vi "feedback(Host)_PIDXYZ_laserPID_COMTEMP.vi"(5 "RIO Device":T2="RIO0") -> ()   [LabVIEW 2018]
doc: "This VI will will initialize the FPGA VI and then continually read and convert single point values from 4 channels of an analog input module."
uses:
  <vilib>/userdefined/High Color/nirio_resource_hc.ctl
  <vilib>/rvi/Analysis/host/Butterworth/config/Butterworth Filter Order.ctl
  <vilib>/rvi/Analysis/host/Butterworth/config/Butterworth Filter Type.ctl
  <vilib>/FPGAPlugInAG/PXIe-7856R/niLvFpga_Open_PXIe-7856R.vi
  <vilib>/FPGAPlugInAG/PXIe-7856R/niLvFpga_Run_PXIe-7856R.vi
  <vilib>/Utility/error.llb/Error Cluster From Error Code.vi
  <vilib>/rvi/errors/niLvFpgaAdjustHostInterfaceError.vi
  <vilib>/rvi/Analysis/host/Butterworth/config/BwScaledCoefficients.vi
  <vilib>/rvi/Analysis/host/Notch/config/NotchScaledCoefficients.vi
  <vilib>/Utility/file.llb/Read From Spreadsheet File (I64).vi
  <vilib>/FPGAPlugInAG/PXIe-7856R/niLvFpga_Close_PXIe-7856R.vi
  <vilib>/rvi/interface/nirviOpenFPGA/nirviOpenFPGA.xnode
  FPGA Bitfiles/Microspherefeedb_FPGATarget2_(FPGA)PIDXYZ_reset_voltage.lvbitx
  <vilib>/rvi/interface/nirviMethod/nirviMethod.xnode
  <vilib>/rvi/interface/nirviReadWriteControl/nirviReadWriteControl.xnode
  <vilib>/rvi/Analysis/host/Butterworth/XNode/ButterworthCoefficients.xnode
  <vilib>/rvi/Analysis/host/Notch/XNode/NotchCoefficients.xnode
  <vilib>/rvi/interface/nirviCloseFPGA/nirviCloseFPGA.xnode
  <vilib>/rvi/Analysis/host/Public/NI_FpgaMspHost.lvlib
  NiFpgaLv.dll
panel:
  in  "Reset voltage":bool
  in  "If revert AO4 and AO5":bool
  in  "notch Q factor2 y":dbl=1.27
  in  "notch frequency2 y":dbl=265.5
  in  "If scan frequency (AO6 and AO7)?":bool
  in  "Amplitude AO7":i16
  in  "Amplitude AO6":i16
  in  "Amplitude AO5":i16
  in  "Amplitude AO4":i16
  in  "reset AO7":bool=TRUE
  in  "frequency AO7(Hz)":dbl=200000.0
  in  "phase offset AO7":fxp<+,32,0>
  in  "reset AO6":bool=TRUE
  in  "frequency AO6(Hz)":dbl=100000.0
  in  "phase offset AO6":fxp<+,32,0>=0.75
  in  "reset AO5":bool=TRUE
  in  "frequency AO5(Hz)":dbl=87.0
  in  "phase offset AO5":fxp<+,32,0>
  in  "reset AO4":bool=TRUE
  in  "frequency AO4(Hz)":dbl
  in  "phase offset AO4":fxp<+,32,0>
  in  "notch Q factor1 y":dbl=1.27
  in  "notch Q factor x":dbl=5.0
  in  "notch frequency1 y":dbl=572.4
  in  "notch frequency x":dbl=1000.0
  out "accum out z2":dbl(graph)
  out "accum out z1":dbl(graph)=1111.0
  in  "Reset x accum":bool=TRUE
  in  "Reset y accum":bool=TRUE
  in  "Reset z accum":bool=TRUE
  in  "Big Number":sgl=10000.0
  in  "amplitude_sine_EOM (V)":sgl
  in  "Freqency_sine_EOM (Hz)":sgl
  in  "Cluster":T1={"activate COMx"=FALSE, "activate  COMy"=FALSE, "activate COMz"=FALSE, "frequency (kHz)"=0.001500000013038516, "duty cycle (periods)"=0.10000000009313226, "offset"=8192, "amplitude"=8192, "Pz?"=FALSE, "Y_emergency_threshould"=23000, "X_emergency_threshould"=23000, "No_integral_Gain"=FALSE}
  in  "LP FF Z before":dbl=5000.0
  in  "LP FF Y before":dbl=5000.0
  in  "LP FF X Before":dbl=5000.0
  in  "LP FF Z":dbl=4200.0
  in  "LP FF Y":dbl=1300.0
  in  "LP FF X":dbl=1300.0
  in  "Lower lim Y before":fxp<+/-,16,16>=-150.0
  in  "Upper lim Y before":fxp<+/-,16,16>=150.0
  in  "Lower lim X before":fxp<+/-,16,16>=-15000.0
  in  "Upper lim X before":fxp<+/-,16,16>=15000.0
  in  "?":u16(ring)=2 items=["Both", "AOD", "Bead"]
  in  "?":u16(ring)=2 items=["Both", "AOD", "Bead"]
  out "Tot feedback + DC, Z":i16(graph)=5000
  out "Individual feedback, Z":cluster{"fb_0":i16, "fb_d0":i16}(graph)
  out "AI 2":cluster{"AI1":i16, "AI4":i16}(graph)={"AI1"=-2580, "AI4"=-2580}
  in  "Use PID Y before":bool
  in  "Use PID X before":bool
  in  "Ig Y before":fxp<+/-,24,-4>
  in  "Dg Y before":fxp<+/-,24,12>
  in  "Pg Y before":fxp<+/-,24,12>
  in  "Ig X before":fxp<+/-,24,-4>
  in  "Dg X before":fxp<+/-,24,12>
  in  "Pg X before":fxp<+/-,24,12>
  in  "Y before setpoint":i16
  in  "X before setpoint":i16
  in  "dg band X before":fxp<+/-,24,12>
  in  "dg band Y before":fxp<+/-,24,12>
  in  "hp freq X band before":dbl=5000.0
  in  "lp freq X band before":dbl=5000.0
  in  "hp freq X before":dbl=5000.0
  in  "lp freq X before":dbl=5000.0
  in  "hp freq Y band before":dbl=5000.0
  in  "lp freq Y band before":dbl=5000.0
  in  "hp freq Y before":dbl=5000.0
  in  "lp freq Y before":dbl=5000.0
  out "EOM_amplitude_out":dbl=-9.299359169972536
  in  "EOM_offset (-10 to 10 V)":dbl
  in  "EOM_amplitude (-10 to 10 V)":dbl=-9.3
  in  "EOM_threshold (0 to 1), (2*thr - 1)*ampli":dbl
  in  "EOM reset":bool
  in  "hp freq band Z before":dbl=5000.0
  in  "lp freq band Z before":dbl=5000.0
  in  "dg band Z before":fxp<+/-,24,12>
  in  "hp freq bandZ":dbl=49.0
  in  "lp freq bandZ":dbl=45.0
  in  "dg band Z":fxp<+/-,24,12>
  in  "dg band Y":fxp<+/-,24,12>
  in  "hp freq bandY":dbl=5000.0
  in  "lp freq bandY":dbl=5000.0
  in  "hp freq bandX":dbl=5000.0
  in  "lp freq bandX":dbl=5000.0
  in  "dg band X":fxp<+/-,24,12>
  in  "Pg Y":fxp<+/-,24,12>
  in  "Ig Y":fxp<+/-,24,-4>=8.009374141693115e-07
  in  "Pg X":fxp<+/-,24,12>
  in  "Ig X":fxp<+/-,24,-4>=-8.009374141693115e-07
  in  "End value arb (ch1)":fxp<+/-,32,16>
  in  "Step arb (ch1)":fxp<+/-,32,16>=0.100006103515625
  in  "Arb gain (Z)":fxp<+/-,24,12>
  in  "z arb scale":fxp<+/-,33,17>
  in  "ramp arb drive":bool
  in  "End value arb (ch0)":fxp<+/-,32,16>
  in  "Step arb (ch0)":fxp<+/-,32,16>
  in  "Delay Time (s) arb":dbl=0.001 caption="Delay Time (s)"
  in  "Buffer file path":path=path "C:/Users/yalem/GitHub/Documents/Optlev/scriptssinx_buffer.txt"
  in  "Write data to buffers":bool
  in  "Arb steps per cycle":u16=2
  in  "Arb gain (Y)":fxp<+/-,24,12>
  in  "Arb gain (X)":fxp<+/-,24,12>
  in  "Z before setpoint":i16
  in  "Upper lim Z before":fxp<+/-,16,16>=9999.0
  in  "Lower lim Z before":fxp<+/-,16,16>=-10000.0
  in  "hp freq Z before":dbl=5000.0
  in  "lp freq Z before":dbl=5000.0
  in  "Use PID Z before":bool
  in  "hp freq Y":dbl=400.0
  in  "hp freq X":dbl=400.0
  in  "lp freq X":dbl=200.0
  in  "DC offset X":i16=23000
  in  "Lower lim X":fxp<+/-,16,16>=-15000.0
  in  "Upper lim X":fxp<+/-,16,16>=15000.0
  in  "Dg X":fxp<+/-,24,12>
  in  "X setpoint":i16
  in  "change pars":bool
  in  "hp freq Z":dbl=4200.0
  in  "lp freq Y":dbl=200.0
  in  "lp freq Z":dbl=4200.0
  in  "ramp power":bool
  in  "End value power":i16=3000
  in  "Step power":i16=30
  in  "Delay Time (s) power":dbl=0.05 caption="Delay Time (s)"
  in  "Count(usec)":u32=10
  in  "?":u16(ring)=2 items=["Both", "AOD", "Bead"]
  in  "?":u16(ring)=2 items=["Both", "AOD", "Bead"]
  in  "?":u16(ring)=2 items=["Both", "AOD", "Bead"]
  in  "?":u16(ring)=2 items=["Both", "AOD", "Bead"]
  in  "Pg Z before":fxp<+/-,24,12>
  in  "Ig Z before":fxp<+/-,24,-4>
  in  "Dg Z before":fxp<+/-,24,12>
  in  "Ig Z":fxp<+/-,24,-4>=2.0116567611694336e-07
  in  "DC offset Z":i16=25000
  in  "Lower lim Z":fxp<+/-,16,16>=-22500.0
  in  "Upper lim Z":fxp<+/-,16,16>=23000.0
  in  "Dg Z":fxp<+/-,24,12>
  in  "Pg Z":fxp<+/-,24,12>
  in  "Z setpoint":i16=-3700
  in  "change pars 2":bool
  in  "change pars 1":bool
  in  "DC offset Y":i16=15000
  in  "Lower lim Y":fxp<+/-,16,16>=-20000.0
  in  "Upper lim Y":fxp<+/-,16,16>=20000.0
  in  "Dg Y":fxp<+/-,24,12>
  in  "Y setpoint":i16
  out "Tot feedback + DC, Y":i16(graph)=15000
  out "Individual feedback, Y":cluster{"fb_0":i16, "fb_d0":i16}(graph)
  out "AI1":cluster{"AI1":i16, "AI4":i16}(graph)={"AI1"=678, "AI4"=678}
  out "Tot feedback + DC, X":i16(graph)=23000
  out "Individual feedback, X":cluster{"fb_0":i16, "fb_d0":i16}(graph)
  out "AI0":cluster{"AI0":i16, "AI3":i16}(graph)={"AI0"=32295, "AI3"=32295}
  in  "stop":bool
  # "FPGA feedback GUI"
  # "Bead arbitrary drive:"
  # "PID controls, X (ch 0):"
  # "Bead feedback:"
  # "PID controls, Y (ch 1):"
  # "Bead feedback:"
  # "Rotation Control"
  # "AO6: Front\nAO7: Window\nAO4: Back\nAO5: Top"
  # "(mV)"
  # "Phase is in unit of periods"
  # "PID controls, Z (ch 2):"
  # "Bead feedback:"
  # "AOD feeback:"
types:
  T1 = cluster{"activate COMx":bool, "activate  COMy":bool, "activate COMz":bool, "frequency (kHz)":fxp<+,32,0>, "duty cycle (periods)":fxp<+,32,0>, "offset":i16, "amplitude":i16, "Pz?":bool, "Y_emergency_threshould":i16, "X_emergency_threshould":i16, "No_integral_Gain":bool}
  T2 = typedef "nirio_resource_hc.ctl" = tag
  T3 = cluster{"AI X plot":i16, "AI X before chamber plot":i16}
  T4 = cluster{"AI X before chamber plot":i16, "AI X before chamber plot":i16}
  T5 = cluster{"fb X plot":i16, "fb X before chamber plot":i16}
  T6 = cluster{"fb X before chamber plot":i16, "fb X before chamber plot":i16}
  T7 = cluster{"AI Y plot":i16, "AI Y before chamber plot":i16}
  T8 = cluster{"AI Y before chamber plot":i16, "AI Y before chamber plot":i16}
  T9 = cluster{"fb Y plot":i16, "fb Y before chamber plot":i16}
  T10 = cluster{"fb Y before chamber plot":i16, "fb Y before chamber plot":i16}
  T11 = cluster{"AI Z plot":i16, "AI Z before chamber plot":i16}
  T12 = cluster{"AI Z before chamber plot":i16, "AI Z before chamber plot":i16}
  T13 = cluster{"fb Z plot":i16, "fb Z before chamber plot":i16}
  T14 = cluster{"fb Z before chamber plot":i16, "fb Z before chamber plot":i16}
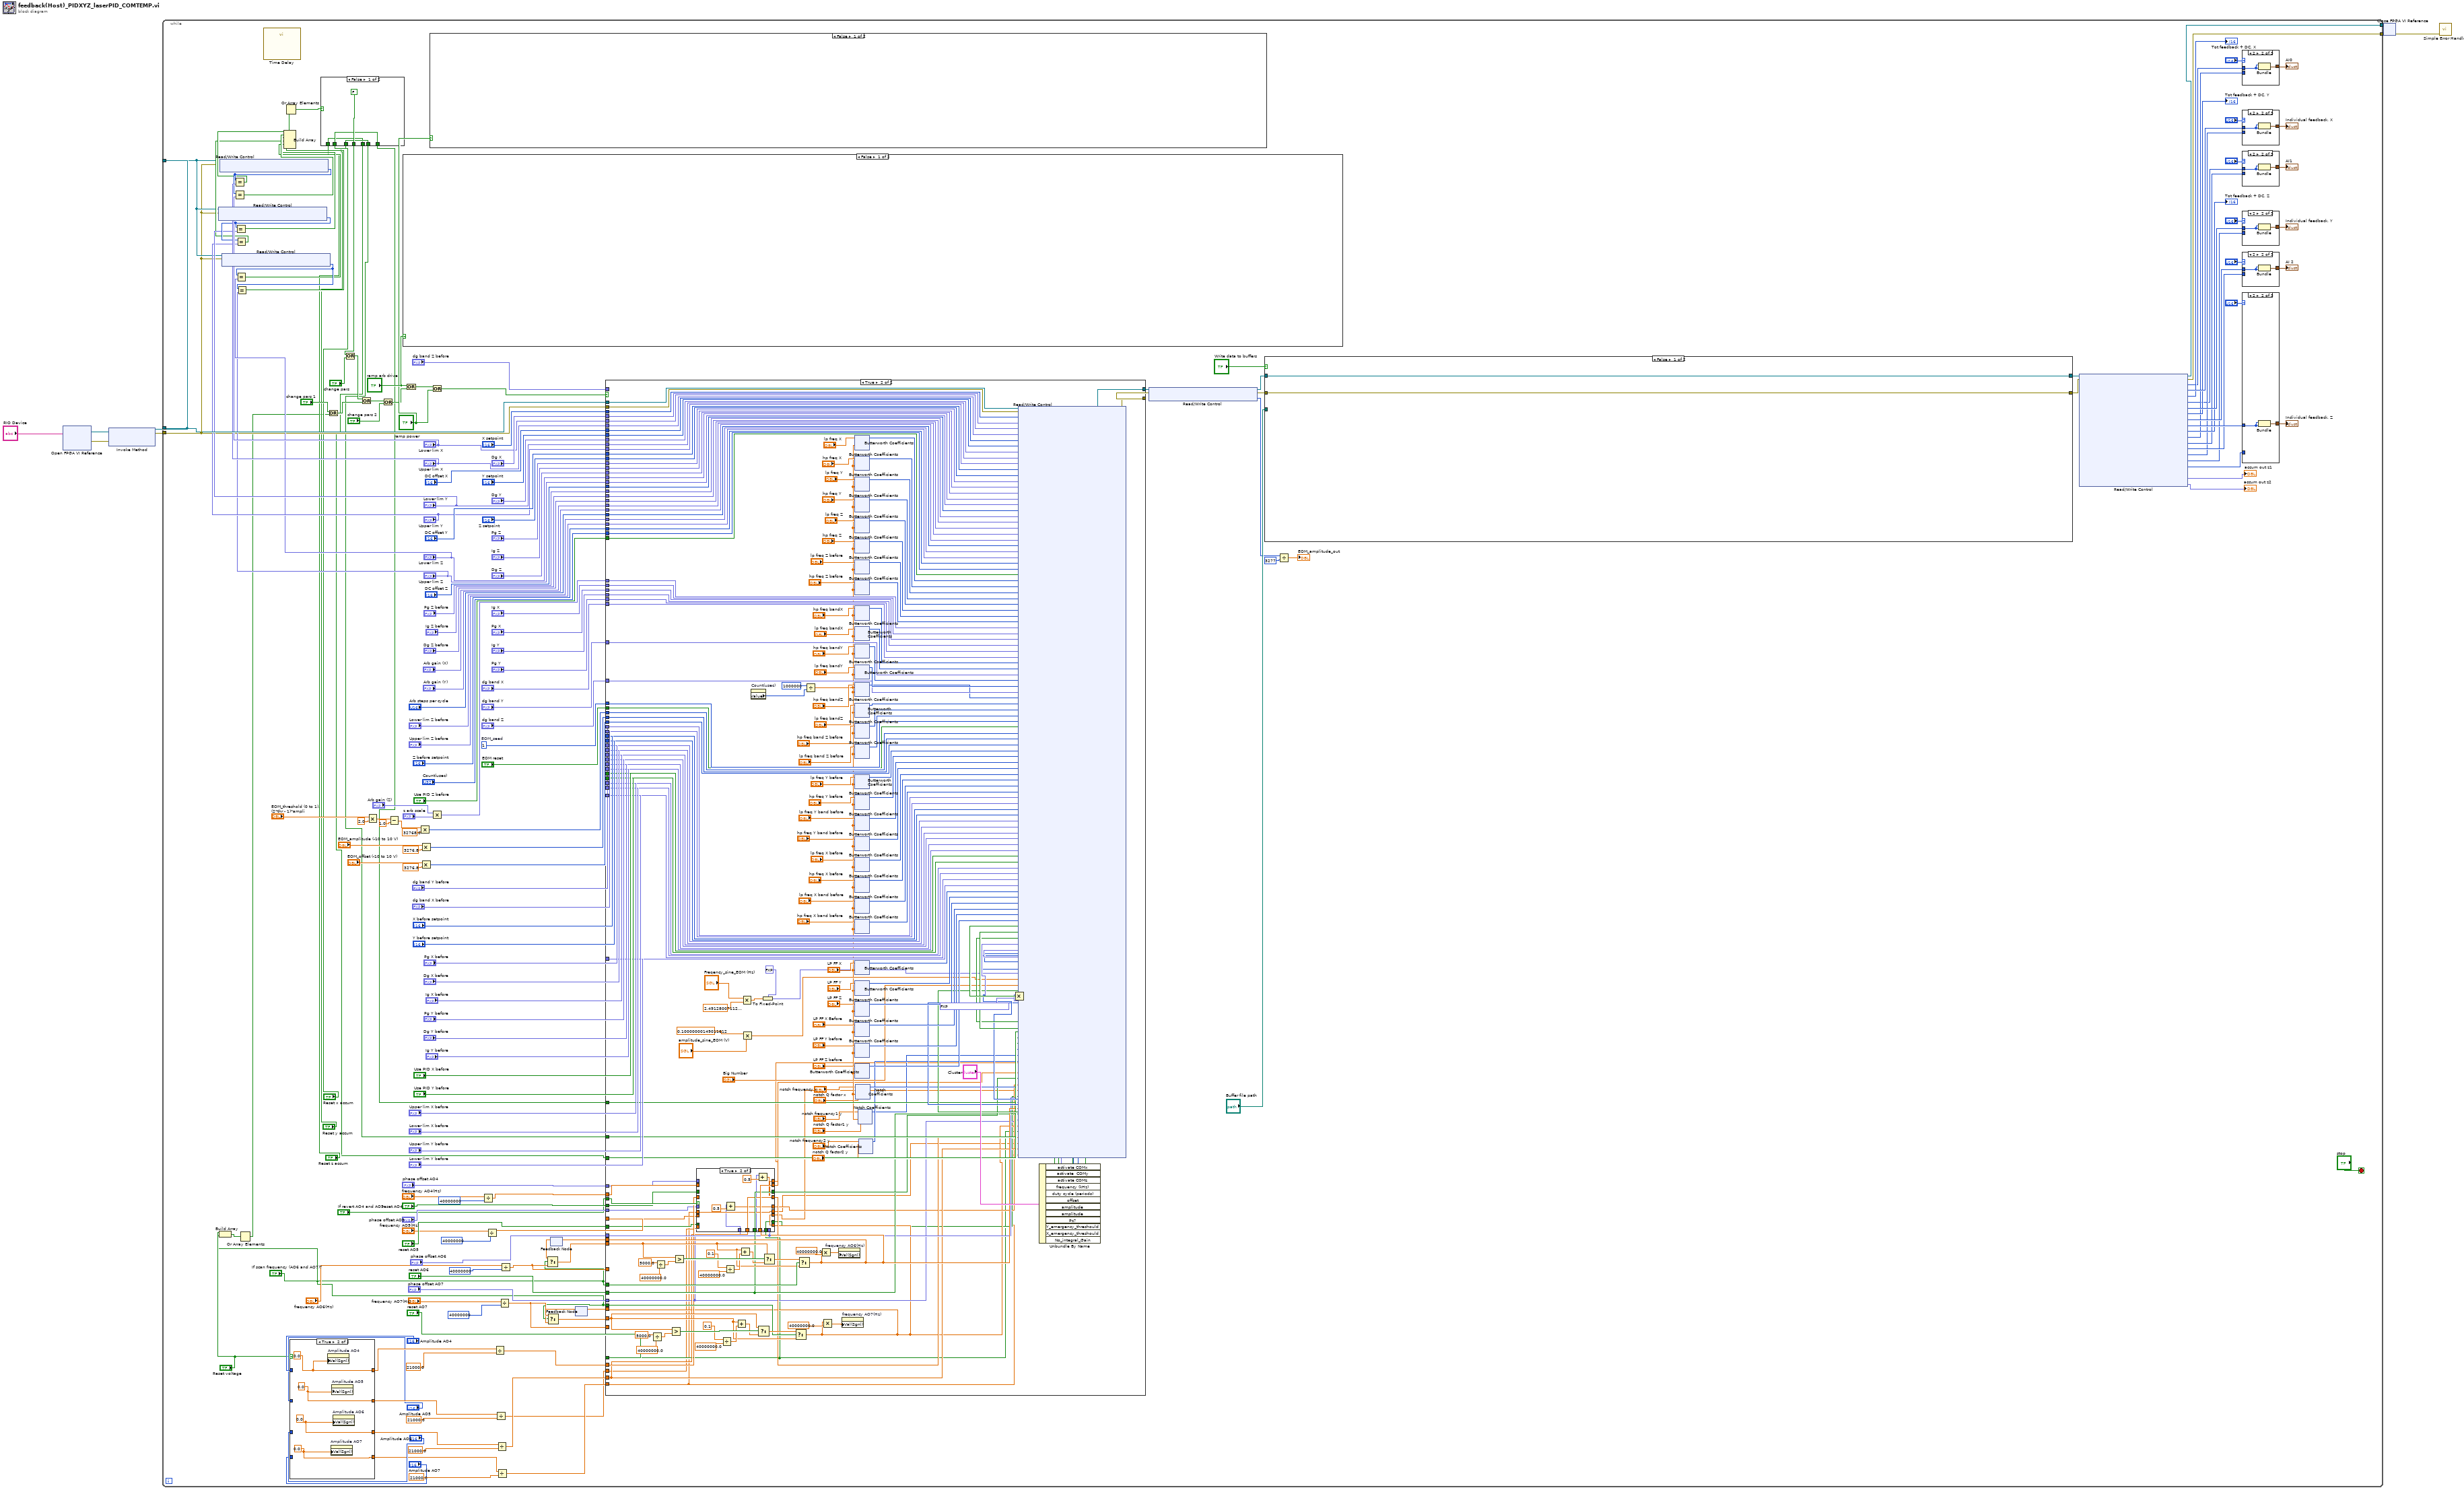
[diagram p0: block diagram]
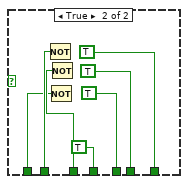
[diagram p3: hidden frame]
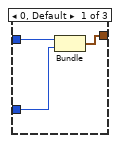
[diagram p4: hidden frame]
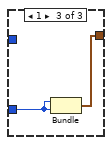
[diagram p5: hidden frame]
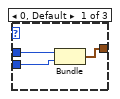
[diagram p6: hidden frame]
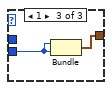
[diagram p7: hidden frame]
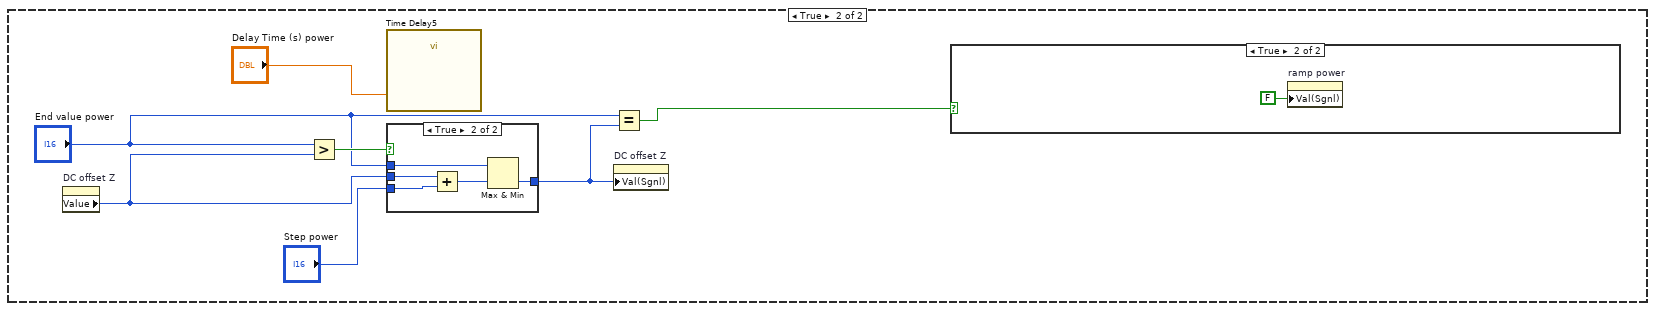
[diagram p8: hidden frame]
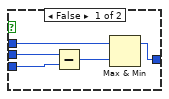
[diagram p10: hidden frame]
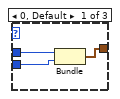
[diagram p11: hidden frame]
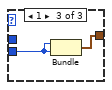
[diagram p12: hidden frame]
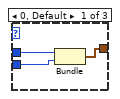
[diagram p13: hidden frame]
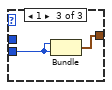
[diagram p14: hidden frame]
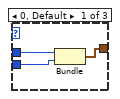
[diagram p15: hidden frame]
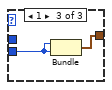
[diagram p16: hidden frame]
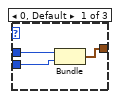
[diagram p17: hidden frame]
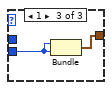
[diagram p18: hidden frame]
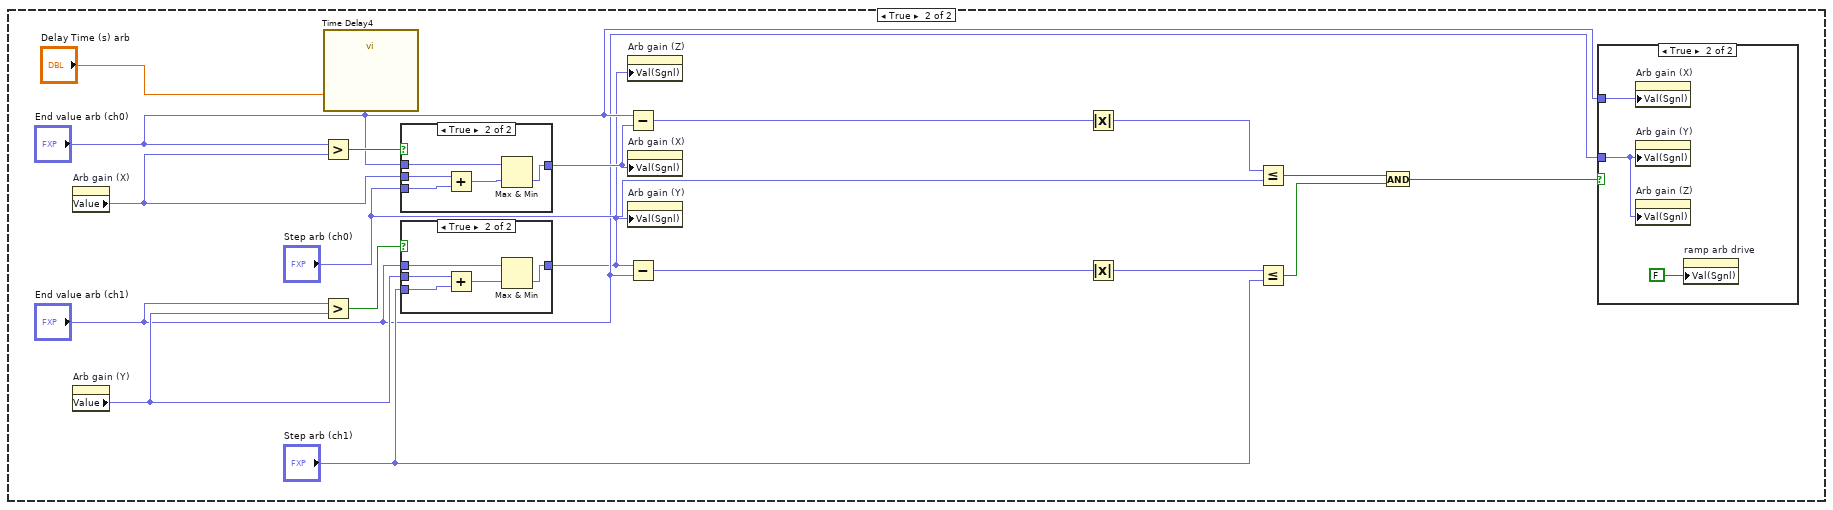
[diagram p19: hidden frame]
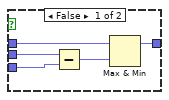
[diagram p20: hidden frame]
diagram:
  n1 = xnode "Open FPGA VI Reference"("resource name"="RIO Device") -> ("FPGA VI Reference Out"=w5:refnum<k20>, "error out"=w4:errorcluster)  [unwired: 1 in]
  n2 = xnode "Invoke Method"("FPGA VI Reference In"=w5, "error in"=w4) -> ("FPGA VI Reference Out"=w1:refnum<k20>, "error out"=w6:errorcluster)  [unwired: 1 in]
  n3 = while {
    tunnel: w1 -> [w196]
    tunnel: w6 -> [w45]
    tunnel: [w89] -> w3
    tunnel: [w88] -> w2
    tunnel: w1 -> [w46]
    stop <- "stop" stop-if-true
    w144 = u32 1  # EOM_seed
    n4 = xnode "Read/Write Control"("FPGA VI Reference In"=w46, "error in"=w45) -> ("fb Y plot"=w57:i16)  [unwired: 2 out]
    n5 = Build Array("If scan frequency (AO6 and AO7)?", "Reset voltage") -> (w12:bool[])
    n6 = xnode "Read/Write Control"("FPGA VI Reference In"=w46, "error in"=w45) -> ("fb X plot"=w62:i16)  [unwired: 2 out]
    n7 = xnode "Read/Write Control"("FPGA VI Reference In"=w46, "error in"=w45) -> ("fb Z plot"=w52:i16)  [unwired: 2 out]
    n8 = Equal?(x=w62, y="Upper lim X") -> (x = y?=w60:bool)
    n9 = Equal?(x=w62, y="Lower lim X") -> (x = y?=w59:bool)
    n10 = Equal?(x=w57, y="Lower lim Y") -> (x = y?=w54:bool)
    n11 = Equal?(x=w57, y="Upper lim Y") -> (x = y?=w53:bool)
    n12 = Equal?(x=w52, y="Lower lim Z") -> (x = y?=w49:bool)
    n13 = Equal?(x=w52, y="Upper lim Z") -> (x = y?=w48:bool)
    n14 = Or Array Elements(Boolean array=w12) -> (logical OR=w10:bool)
    n15 = call "Time Delay"() -> ()  [unwired: 11 in, 1 out]
    n16 = Build Array(w60, w59, w54, w53, w49, w48) -> (w58:bool[])
    n17 = Or Array Elements(Boolean array=w58) -> (logical OR=w47:bool)
    n18 = case shown="True" "Reset voltage" {
      tunnel: "Amplitude AO4" -> [w204 _]
      tunnel: [w204 w208] -> w20
      tunnel: [w203 w207] -> w19
      tunnel: "Amplitude AO5" -> [w203 _]
      tunnel: [w202 w206] -> w17
      tunnel: "Amplitude AO6" -> [w202 _]
      tunnel: "Amplitude AO7" -> [w201 _]
      tunnel: [w201 w205] -> w14
      frame False {
      }
      frame True {
        w205 = 0.0
        w206 = 0.0
        w207 = 0.0
        w208 = 0.0
        n19 = property on="Amplitude AO4" class="DigNum (strict)"("Val(Sgnl)"=w208) -> ()  [unwired: 2 in, 2 out]
        n20 = property on="Amplitude AO7" class="DigNum (strict)"("Val(Sgnl)"=w205) -> ()  [unwired: 2 in, 2 out]
        n21 = property on="Amplitude AO5" class="DigNum (strict)"("Val(Sgnl)"=w207) -> ()  [unwired: 2 in, 2 out]
        n22 = property on="Amplitude AO6" class="DigNum (strict)"("Val(Sgnl)"=w206) -> ()  [unwired: 2 in, 2 out]
      }
    }
    n23 = case shown="False" w47 {
      tunnel: [FALSE TRUE] -> w42
      tunnel: [w211 TRUE] -> w41
      tunnel: "Reset x accum" -> [w211 w218]
      tunnel: "Reset y accum" -> [w210 w217]
      tunnel: [w210 TRUE] -> w38
      tunnel: "Reset z accum" -> [w209 w216]
      tunnel: [w209 TRUE] -> w36
      frame False {
      }
      frame True {
        n24 = Not(x=w218) -> ()  [unwired: 1 out]
        n25 = Not(x=w216) -> ()  [unwired: 1 out]
        n26 = Not(x=w217) -> ()  [unwired: 1 out]
      }
    }
    n27 = Or(x="change pars 1", y=w10) -> (x .or. y?=w75:bool)
    n28 = Or(x=w42, y="change pars") -> (x .or. y?=w44:bool)
    n29 = Or(x=w44, y=w75) -> (x .or. y?=w178:bool)
    n30 = Multiply(x="EOM_threshold (0 to 1), (2*thr - 1)*ampli", y=2.0) -> (x*y=w140:dbl)
    n31 = Or(x=w178, y="change pars 2") -> (x .or. y?=w157:bool)
    n32 = Subtract(x=w140, y=1.0) -> (x-y=w138:dbl)
    n33 = case shown="False" "ramp arb drive" {
      frame False {
      }
      frame True {
        n34 = property on="Arb gain (X)" class="DigNum (strict)"() -> ("Value"=w296:fxp<+/-,24,12>)  [unwired: 2 in, 2 out]
        n35 = property on="Arb gain (Y)" class="DigNum (strict)"() -> ("Value"=w293:fxp<+/-,24,12>)  [unwired: 2 in, 2 out]
        n36 = Greater?(x="End value arb (ch0)", y=w296) -> (0:w297:bool)
        n37 = Greater?(x="End value arb (ch1)", y=w293) -> (0:w294:bool)
        n38 = call "Time Delay4"("Delay Time (s)"="Delay Time (s) arb") -> ()  [unwired: 10 in, 1 out]
        n39 = case shown="True" w297 {
          tunnel: "End value arb (ch0)" -> [w312 w317]
          tunnel: w296 -> [w315 w320]
          tunnel: "Step arb (ch0)" -> [w314 w319]
          tunnel: [w311 w316] -> w292
          frame False {
            n40 = Subtract(x=w315, y=w314) -> (x-y=w313:fxp<+/-,33,17>)
            n41 = Max & Min(x=w312, y=w313) -> (max(x,y)=w311:fxp<+/-,33,17>)  [unwired: 1 out]
          }
          frame True {
            n42 = Add(x=w320, y=w319) -> (x+y=w318:fxp<+/-,33,17>)
            n43 = Max & Min(x=w317, y=w318) -> (min(x,y)=w316:fxp<+/-,33,17>)  [unwired: 1 out]
          }
        }
        n44 = case shown="True" w294 {
          tunnel: "End value arb (ch1)" -> [w299 w305]
          tunnel: w293 -> [w302 w303]
          tunnel: "Step arb (ch1)" -> [w301 w307]
          tunnel: [w298 w304] -> w280
          frame False {
            n45 = Subtract(x=w302, y=w301) -> (x-y=w300:fxp<+/-,33,17>)
            n46 = Max & Min(x=w299, y=w300) -> (max(x,y)=w298:fxp<+/-,33,17>)  [unwired: 1 out]
          }
          frame True {
            n47 = Add(x=w303, y=w307) -> (x+y=w306:fxp<+/-,33,17>)
            n48 = Max & Min(x=w305, y=w306) -> (min(x,y)=w304:fxp<+/-,33,17>)  [unwired: 1 out]
          }
        }
        n49 = property on="Arb gain (Z)" class="DigNum (strict)"("Val(Sgnl)"=w280) -> ()  [unwired: 2 in, 2 out]
        n50 = Subtract(x="End value arb (ch0)", y=w292) -> (x-y=w291:fxp<+/-,34,18>)
        n51 = property on="Arb gain (X)" class="DigNum (strict)"("Val(Sgnl)"=w292) -> ()  [unwired: 2 in, 2 out]
        n52 = property on="Arb gain (Y)" class="DigNum (strict)"("Val(Sgnl)"=w280) -> ()  [unwired: 2 in, 2 out]
        n53 = Subtract(x=w280, y="End value arb (ch1)") -> (x-y=w288:fxp<+/-,34,18>)
        n54 = Absolute Value(x=w291) -> (abs(x)=w290:fxp<+,33,17>)
        n55 = Absolute Value(x=w288) -> (abs(x)=w287:fxp<+,33,17>)
        n56 = Less Or Equal?(x=w290, y="Step arb (ch0)") -> (x <= y?=w284:bool)
        n57 = Less Or Equal?(x=w287, y="Step arb (ch1)") -> (x <= y?=w283:bool)
        n58 = And(x=w284, y=w283) -> (x .and. y?=w285:bool)
        n59 = case shown="True" w285 {
          tunnel: "End value arb (ch0)" -> [_ w309]
          tunnel: "End value arb (ch1)" -> [_ w308]
          frame False {
          }
          frame True {
            n60 = property on="Arb gain (X)" class="DigNum (strict)"("Val(Sgnl)"=w309) -> ()  [unwired: 2 in, 2 out]
            n61 = property on="Arb gain (Y)" class="DigNum (strict)"("Val(Sgnl)"=w308) -> ()  [unwired: 2 in, 2 out]
            n62 = property on="Arb gain (Z)" class="DigNum (strict)"("Val(Sgnl)"=w308) -> ()  [unwired: 2 in, 2 out]
            n63 = property on="ramp arb drive" class="Bool (strict)"("Val(Sgnl)"=FALSE) -> ()  [unwired: 2 in, 2 out]
          }
        }
      }
    }
    n64 = Or(x="ramp arb drive", y=w157) -> (x .or. y?=w164:bool)
    n65 = Multiply(x=w138, y=32768.0) -> (x*y=w136:i16)
    n66 = Multiply(x="EOM_amplitude (-10 to 10 V)", y=3276.8) -> (x*y=w133:i16)
    n67 = Multiply(x="EOM_offset (-10 to 10 V)", y=3276.8) -> (x*y=w130:i16)
    n68 = case shown="False" "ramp power" {
      frame False {
      }
      frame True {
        n69 = property on="DC offset Z" class="DigNum (strict)"() -> ("Value"=w235:i16)  [unwired: 2 in, 2 out]
        n70 = Greater?(x="End value power", y=w235) -> (0:w240:bool)
        n71 = call "Time Delay5"("Delay Time (s)"="Delay Time (s) power") -> ()  [unwired: 10 in, 1 out]
        n72 = case shown="True" w240 {
          tunnel: "End value power" -> [w243 w248]
          tunnel: w235 -> [w246 w251]
          tunnel: "Step power" -> [w245 w250]
          tunnel: [w242 w247] -> w234
          frame False {
            n73 = Subtract(x=w246, y=w245) -> (x-y=w244:i16)
            n74 = Max & Min(x=w243, y=w244) -> (max(x,y)=w242:i16)  [unwired: 1 out]
          }
          frame True {
            n75 = Add(x=w251, y=w250) -> (x+y=w249:i16)
            n76 = Max & Min(x=w248, y=w249) -> (min(x,y)=w247:i16)  [unwired: 1 out]
          }
        }
        n77 = Equal?(x="End value power", y=w234) -> (x = y?=w239:bool)
        n78 = property on="DC offset Z" class="DigNum (strict)"("Val(Sgnl)"=w234) -> ()  [unwired: 2 in, 2 out]
        n79 = case shown="True" w239 {
          frame False {
          }
          frame True {
            n80 = property on="ramp power" class="Bool (strict)"("Val(Sgnl)"=FALSE) -> ()  [unwired: 2 in, 2 out]
          }
        }
      }
    }
    n81 = Or(x=w164, y="ramp power") -> (x .or. y?=w90:bool)
    n82 = Multiply(x="Arb gain (Z)", y="z arb scale") -> (x*y=w154:fxp<+/-,56,28>)
    n83 = Divide(x="frequency AO4(Hz)", y=40000000) -> (x/y=w83:dbl)
    n84 = Divide(x="frequency AO5(Hz)", y=40000000) -> (x/y=w82:dbl)
    n85 = Divide(x=w20, y=21000.0) -> (x/y=w64:dbl)
    n86 = Divide(x=w19, y=21000.0) -> (x/y=w65:dbl)
    n87 = Divide(x=w17, y=21000.0) -> (x/y=w66:dbl)
    n88 = Divide(x=w14, y=21000.0) -> (x/y=w70:dbl)
    n89 = Divide(x="frequency AO7(Hz)", y=40000000) -> (x/y=w72:dbl)
    n90 = Divide(x="frequency AO6(Hz)", y=40000000) -> (x/y=w77:dbl)
    n91 = feedback #1() -> (w78:dbl)  [unwired: 1 in]
    n92 = Select(t=w78, s="If scan frequency (AO6 and AO7)?", f=w77) -> (s? t:f=w29:dbl)
    n93 = feedback #2() -> (w73:dbl)  [unwired: 1 in]
    n94 = Select(t=w73, s="If scan frequency (AO6 and AO7)?", f=w72) -> (s? t:f=w28:dbl)
    n95 = case shown="True" w90 {
      tunnel: w45 -> [w404 w606]
      tunnel: [w404 w614] -> w129
      tunnel: [w403 w613] -> w128
      tunnel: "X setpoint" -> [_ w612]
      tunnel: "Dg X" -> [_ w611]
      tunnel: "Upper lim X" -> [_ w609]
      tunnel: "Lower lim X" -> [_ w610]
      tunnel: "DC offset X" -> [_ w608]
      tunnel: w196 -> [w403 w607]
      tunnel: "Y setpoint" -> [_ w605]
      tunnel: "Dg Y" -> [_ w604]
      tunnel: "Lower lim Y" -> [_ w603]
      tunnel: "Upper lim Y" -> [_ w602]
      tunnel: "DC offset Y" -> [_ w601]
      tunnel: "Z setpoint" -> [_ w600]
      tunnel: "Pg Z" -> [_ w599]
      tunnel: "Ig Z" -> [_ w598]
      tunnel: "Dg Z" -> [_ w597]
      tunnel: "Lower lim Z" -> [_ w596]
      tunnel: "Upper lim Z" -> [_ w595]
      tunnel: "DC offset Z" -> [_ w594]
      tunnel: "Pg Z before" -> [_ w593]
      tunnel: "Ig Z before" -> [_ w592]
      tunnel: "Dg Z before" -> [_ w537]
      tunnel: "Arb gain (Y)" -> [_ w578]
      tunnel: "Arb steps per cycle" -> [_ w591]
      tunnel: "Count(usec)" -> [_ w590]
      tunnel: "Use PID Z before" -> [_ w581]
      tunnel: "Lower lim Z before" -> [_ w577]
      tunnel: "Upper lim Z before" -> [_ w576]
      tunnel: "Z before setpoint" -> [_ w575]
      tunnel: w154 -> [_ w566]
      tunnel: "Ig X" -> [_ w565]
      tunnel: "Pg X" -> [_ w564]
      tunnel: "Ig Y" -> [_ w563]
      tunnel: "Pg Y" -> [_ w562]
      tunnel: "dg band X" -> [_ w561]
      tunnel: "dg band Y" -> [_ w554]
      tunnel: "dg band Z" -> [_ w551]
      tunnel: "dg band Z before" -> [_ _]
      tunnel: w144 -> [_ w542]
      tunnel: "EOM reset" -> [_ w541]
      tunnel: w136 -> [_ w540]
      tunnel: w133 -> [_ w539]
      tunnel: w130 -> [_ w538]
      tunnel: "dg band Y before" -> [_ w520]
      tunnel: "dg band X before" -> [_ w519]
      tunnel: "X before setpoint" -> [_ w518]
      tunnel: "Y before setpoint" -> [_ w517]
      tunnel: "Pg X before" -> [_ w516]
      tunnel: "Dg X before" -> [_ w515]
      tunnel: "Ig X before" -> [_ w514]
      tunnel: "Pg Y before" -> [_ w513]
      tunnel: "Dg Y before" -> [_ w512]
      tunnel: "Ig Y before" -> [_ w511]
      tunnel: "Use PID X before" -> [_ w510]
      tunnel: "Use PID Y before" -> [_ w509]
      tunnel: "Upper lim X before" -> [_ w508]
      tunnel: "Lower lim X before" -> [_ w507]
      tunnel: "Upper lim Y before" -> [_ w506]
      tunnel: "Lower lim Y before" -> [_ w505]
      tunnel: "Arb gain (X)" -> [_ w492]
      tunnel: w36 -> [_ w468]
      tunnel: w38 -> [_ w467]
      tunnel: w41 -> [_ w466]
      tunnel: "phase offset AO4" -> [_ w422]
      tunnel: w83 -> [_ w429]
      tunnel: "reset AO4" -> [_ w425]
      tunnel: "phase offset AO5" -> [_ w416]
      tunnel: w82 -> [_ w413]
      tunnel: "reset AO5" -> [_ w410]
      tunnel: "phase offset AO6" -> [_ w420]
      tunnel: w29 -> [_ w448]
      tunnel: "reset AO6" -> [_ w423]
      tunnel: "phase offset AO7" -> [_ w414]
      tunnel: w28 -> [_ w436]
      tunnel: "reset AO7" -> [_ w408]
      tunnel: w64 -> [_ w419]
      tunnel: w65 -> [_ w407]
      tunnel: w66 -> [_ w417]
      tunnel: w70 -> [_ w405]
      tunnel: "If scan frequency (AO6 and AO7)?" -> [_ w451]
      tunnel: [w402 w427] -> w79
      tunnel: w77 -> [w402 _]
      tunnel: "If scan frequency (AO6 and AO7)?" -> [_ w437]
      tunnel: [w401 w411] -> w74
      tunnel: w72 -> [w401 _]
      tunnel: "If revert AO4 and AO5" -> [_ w426]
      frame False {
      }
      frame True {
        n96 = Divide(x=5000.0, y=40000000.0) -> (x/y=w447:dbl)
        n97 = Divide(x=5000.0, y=40000000.0) -> (x/y=w459:dbl)
        n98 = Greater?(x=w436, y=w447) -> (0:w444:bool)
        n99 = Greater?(x=w448, y=w459) -> (0:w456:bool)
        n100 = Divide(x=0.1 ("y"), y=40000000.0) -> (x/y=w442:dbl)
        n101 = Divide(x=0.1 ("y"), y=40000000.0) -> (x/y=w454:dbl)
        n102 = Add(x=w436, y=w442) -> (x+y=w438:dbl)
        n103 = Add(x=w448, y=w454) -> (x+y=w449:dbl)
        n104 = Multiply(x="Freqency_sine_EOM (Hz)", y=sgl 2.49128e-08) -> (x*y=w479:sgl)
        n105 = Multiply(x=sgl 0.1, y="amplitude_sine_EOM (V)") -> (x*y=w476:sgl)
        n106 = property on="Count(usec)" class="DigNum (strict)"() -> ("Value"=w586:u32)  [unwired: 2 in, 2 out]
        n107 = Select(t=w436, s=w444, f=w438) -> (s? t:f=w440:dbl)
        n108 = To Fixed-Point(fixed-point type=fxp<+,32,0> 0.0 ("eom sine frequency (periods/tick)"), number=w479) -> (fixed-point=w475:fxp<+,32,0>)
        n109 = Select(t=w448, s=w456, f=w449) -> (s? t:f=w452:dbl)
        n110 = Select(t=w440, s=w437, f=w436) -> (s? t:f=w411:dbl)
        n111 = Select(t=w452, s=w451, f=w448) -> (s? t:f=w427:dbl)
        n112 = case shown="True" w426 {
          tunnel: w429 -> [w622 _]
          tunnel: [w622 w634] -> w428
          tunnel: w427 -> [_ w634]
          tunnel: w425 -> [w621 _]
          tunnel: [w621 w633] -> w424
          tunnel: w423 -> [_ w633]
          tunnel: w422 -> [w620 _]
          tunnel: [w620 w623] -> w421
          tunnel: w420 -> [_ w624]
          tunnel: w419 -> [w619 _]
          tunnel: [w619 w632] -> w418
          tunnel: w417 -> [_ w632]
          tunnel: w416 -> [w618 _]
          tunnel: [w618 w627] -> w415
          tunnel: w414 -> [_ w626]
          tunnel: w413 -> [w617 _]
          tunnel: [w617 w631] -> w412
          tunnel: w411 -> [_ w631]
          tunnel: w410 -> [w616 _]
          tunnel: [w616 w630] -> w409
          tunnel: w408 -> [_ w630]
          tunnel: w407 -> [w615 _]
          tunnel: [w615 w629] -> w406
          tunnel: w405 -> [_ w629]
          frame False {
          }
          frame True {
            n113 = Add(x=w626, y=0.5) -> (x+y=w627:dbl)
            n114 = Add(x=w624, y=0.5) -> (x+y=w623:dbl)
          }
        }
        n115 = Divide(x=u32 1000000, y=w586) -> (x/y=w464:dbl)
        n116 = Multiply(x=w427, y=40000000.0) -> (x*y=w435:dbl)
        n117 = Multiply(x=w411, y=40000000.0) -> (x*y=w434:dbl)
        n118 = property on="frequency AO6(Hz)" class="DigNum (strict)"("Val(Sgnl)"=w435) -> ()  [unwired: 2 in, 2 out]
        n119 = property on="frequency AO7(Hz)" class="DigNum (strict)"("Val(Sgnl)"=w434) -> ()  [unwired: 2 in, 2 out]
        n120 = xnode "Butterworth Coefficients"("cutoff frequency (Hz)"="lp freq X", "sample rate (S/s)"=w464) -> ("scaled coefficients"=w574:i32[])  [unwired: 1 in, 1 out]
        n121 = xnode "Butterworth Coefficients"("cutoff frequency (Hz)"="hp freq X", "sample rate (S/s)"=w464) -> ("scaled coefficients"=w573:i32[])  [unwired: 1 in, 1 out]
        n122 = xnode "Butterworth Coefficients"("cutoff frequency (Hz)"="lp freq Y", "sample rate (S/s)"=w464) -> ("scaled coefficients"=w572:i32[])  [unwired: 1 in, 1 out]
        n123 = xnode "Butterworth Coefficients"("cutoff frequency (Hz)"="hp freq Y", "sample rate (S/s)"=w464) -> ("scaled coefficients"=w571:i32[])  [unwired: 1 in, 1 out]
        n124 = xnode "Butterworth Coefficients"("cutoff frequency (Hz)"="lp freq Z", "sample rate (S/s)"=w464) -> ("scaled coefficients"=w570:i32[])  [unwired: 1 in, 1 out]
        n125 = xnode "Butterworth Coefficients"("cutoff frequency (Hz)"="hp freq Z", "sample rate (S/s)"=w464) -> ("scaled coefficients"=w569:i32[])  [unwired: 1 in, 1 out]
        n126 = xnode "Butterworth Coefficients"("cutoff frequency (Hz)"="lp freq Z before", "sample rate (S/s)"=w464) -> ("scaled coefficients"=w568:i32[])  [unwired: 1 in, 1 out]
        n127 = xnode "Butterworth Coefficients"("cutoff frequency (Hz)"="hp freq Z before", "sample rate (S/s)"=w464) -> ("scaled coefficients"=w567:i32[])  [unwired: 1 in, 1 out]
        n128 = xnode "Butterworth Coefficients"("cutoff frequency (Hz)"="hp freq bandX", "sample rate (S/s)"=w464) -> ("scaled coefficients"=w558:i32[])  [unwired: 1 in, 1 out]
        n129 = xnode "Butterworth Coefficients"("cutoff frequency (Hz)"="lp freq bandX", "sample rate (S/s)"=w464) -> ("scaled coefficients"=w557:i32[])  [unwired: 1 in, 1 out]
        n130 = xnode "Butterworth Coefficients"("cutoff frequency (Hz)"="hp freq bandY", "sample rate (S/s)"=w464) -> ("scaled coefficients"=w552:i32[])  [unwired: 1 in, 1 out]
        n131 = xnode "Butterworth Coefficients"("cutoff frequency (Hz)"="lp freq bandY", "sample rate (S/s)"=w464) -> ("scaled coefficients"=w553:i32[])  [unwired: 1 in, 1 out]
        n132 = xnode "Butterworth Coefficients"("cutoff frequency (Hz)"="hp freq bandZ", "sample rate (S/s)"=w464) -> ("scaled coefficients"=w548:i32[])  [unwired: 1 in, 1 out]
        n133 = xnode "Butterworth Coefficients"("cutoff frequency (Hz)"="lp freq bandZ", "sample rate (S/s)"=w464) -> ("scaled coefficients"=w547:i32[])  [unwired: 1 in, 1 out]
        n134 = xnode "Butterworth Coefficients"("cutoff frequency (Hz)"="hp freq band Z before", "sample rate (S/s)"=w464) -> ("scaled coefficients"=w544:i32[])  [unwired: 1 in, 1 out]
        n135 = xnode "Butterworth Coefficients"("cutoff frequency (Hz)"="lp freq band Z before", "sample rate (S/s)"=w464) -> ("scaled coefficients"=w543:i32[])  [unwired: 1 in, 1 out]
        n136 = xnode "Butterworth Coefficients"("cutoff frequency (Hz)"="lp freq Y before", "sample rate (S/s)"=w464) -> ("scaled coefficients"=w534:i32[])  [unwired: 1 in, 1 out]
        n137 = xnode "Butterworth Coefficients"("cutoff frequency (Hz)"="hp freq Y before", "sample rate (S/s)"=w464) -> ("scaled coefficients"=w533:i32[])  [unwired: 1 in, 1 out]
        n138 = xnode "Butterworth Coefficients"("cutoff frequency (Hz)"="lp freq Y band before", "sample rate (S/s)"=w464) -> ("scaled coefficients"=w530:i32[])  [unwired: 1 in, 1 out]
        n139 = xnode "Butterworth Coefficients"("cutoff frequency (Hz)"="hp freq Y band before", "sample rate (S/s)"=w464) -> ("scaled coefficients"=w529:i32[])  [unwired: 1 in, 1 out]
        n140 = xnode "Butterworth Coefficients"("cutoff frequency (Hz)"="lp freq X before", "sample rate (S/s)"=w464) -> ("scaled coefficients"=w524:i32[])  [unwired: 1 in, 1 out]
        n141 = xnode "Butterworth Coefficients"("cutoff frequency (Hz)"="hp freq X before", "sample rate (S/s)"=w464) -> ("scaled coefficients"=w523:i32[])  [unwired: 1 in, 1 out]
        n142 = xnode "Butterworth Coefficients"("cutoff frequency (Hz)"="lp freq X band before", "sample rate (S/s)"=w464) -> ("scaled coefficients"=w522:i32[])  [unwired: 1 in, 1 out]
        n143 = xnode "Butterworth Coefficients"("cutoff frequency (Hz)"="hp freq X band before", "sample rate (S/s)"=w464) -> ("scaled coefficients"=w521:i32[])  [unwired: 1 in, 1 out]
        n144 = xnode "Butterworth Coefficients"("cutoff frequency (Hz)"="LP FF X", "sample rate (S/s)"=w464) -> ("scaled coefficients"=w503:i32[])  [unwired: 1 in, 1 out]
        n145 = xnode "Butterworth Coefficients"("cutoff frequency (Hz)"="LP FF Y", "sample rate (S/s)"=w464) -> ("scaled coefficients"=w501:i32[])  [unwired: 1 in, 1 out]
        n146 = xnode "Butterworth Coefficients"("cutoff frequency (Hz)"="LP FF Z", "sample rate (S/s)"=w464) -> ("scaled coefficients"=w499:i32[])  [unwired: 1 in, 1 out]
        n147 = xnode "Butterworth Coefficients"("cutoff frequency (Hz)"="LP FF X Before", "sample rate (S/s)"=w464) -> ("scaled coefficients"=w497:i32[])  [unwired: 1 in, 1 out]
        n148 = xnode "Butterworth Coefficients"("cutoff frequency (Hz)"="LP FF Y before", "sample rate (S/s)"=w464) -> ("scaled coefficients"=w495:i32[])  [unwired: 1 in, 1 out]
        n149 = xnode "Butterworth Coefficients"("cutoff frequency (Hz)"="LP FF Z before", "sample rate (S/s)"=w464) -> ("scaled coefficients"=w493:i32[])  [unwired: 1 in, 1 out]
        n150 = xnode "Notch Coefficients"("notch frequency (Hz)"="notch frequency x", "Q factor"="notch Q factor x", "sample rate (S/s)"=w464) -> ("scaled coefficients"=w465:i32[])  [unwired: 1 in, 1 out]
        n151 = xnode "Notch Coefficients"("notch frequency (Hz)"="notch frequency1 y", "Q factor"="notch Q factor1 y", "sample rate (S/s)"=w464) -> ("scaled coefficients"=w430:i32[])  [unwired: 1 in, 1 out]
        n152 = xnode "Notch Coefficients"("notch frequency (Hz)"="notch frequency2 y", "Q factor"="notch Q factor2 y") -> ("scaled coefficients"=w431:i32[])  [unwired: 2 in, 1 out]
        n153 = Unbundle By Name("Cluster") -> ("activate COMx"=w491:bool, "activate  COMy"=w490:bool, "activate COMz"=w489:bool, "frequency (kHz)"=w487:fxp<+,32,0>, "duty cycle (periods)"=w488:fxp<+,32,0>, "offset"=w484:i16, "amplitude"=w483:i16, "Pz?"=w482:bool, "Y_emergency_threshould"=w471:i16, "X_emergency_threshould"=w470:i16, "No_integral_Gain"=w469:bool)  [unwired: 1 out]
        n154 = Multiply(x=w487, y=fxp<+,32,0> 2.491287887096405e-05) -> (x*y=w485:fxp<+,32,0>)
        n155 = xnode "Read/Write Control"("FPGA VI Reference In"=w607, "error in"=w606, "X Setpoint"=w612, "dg X"=w611, "Lower lim X"=w610, "Upper lim X"=w609, "DC offset X"=w608, "Y Setpoint"=w605, "dg Y"=w604, "Lower lim Y"=w603, "Upper lim Y"=w602, "DC offset Y"=w601, "Z Setpoint"=w600, "pg Z"=w599, "ig Z"=w598, "dg Z"=w597, "Lower lim Z"=w596, "Upper lim Z"=w595, "DC offset Z"=w594, "pg Z before"=w593, "ig Z before"=w592, "dg Z before"=w537, "Arb gain (ch0)"=w492, "Arb gain (ch1)"=w578, "Arb steps per cycle"=w591, "Lower lim Z before"=w577, "Upper lim Z before"=w576, "Z before Setpoint"=w575, "Count(uSec)"=w590, "Use Z PID before"=w581, "LP Coeff X"=w574, "HP Coeff X"=w573, "LP Coeff Y"=w572, "HP Coeff Y"=w571, "LP Coeff Z"=w570, "HP Coeff Z"=w569, "LP Coeff band Z before"=w568, "HP coeff band Z before"=w567, "Arb gain (ch2)"=w566, "ig X"=w565, "pg X"=w564, "ig Y"=w563, "pg Y"=w562, "dg band X"=w561, "HP Coeff band X"=w558, "LP Coeff band X"=w557, "dg band Y"=w554, "HP Coeff band Y"=w552, "LP Coeff band Y"=w553, "dg band Z"=w551, "HP Coeff band Z"=w548, "LP Coeff band Z"=w547, "HP Coeff band Z"=w544, "LP Coeff band Z"=w543, "EOM_seed"=w542, "EOM reset"=w541, "EOM_threshold"=w540, "EOM_amplitude"=w539, "EOM_offset"=w538, "LP Coeff Y before"=w534, "HP Coeff Y before"=w533, "LP Coeff band Y before"=w530, "HP coeff band Y before"=w529, "LP Coeff X before"=w524, "HP Coeff X before"=w523, "LP Coeff band X before"=w522, "HP coeff band X before"=w521, "dg band Y before"=w520, "dg band X before"=w519, "X before Setpoint"=w518, "Y before Setpoint"=w517, "pg X before"=w516, "dg X before"=w515, "ig X before"=w514, "pg Y before"=w513, "dg Y before"=w512, "ig Y before"=w511, "Use X PID before"=w510, "Use Y PID before"=w509, "Upper lim X before"=w508, "Lower lim X before"=w507, "Upper lim Y before"=w506, "Lower lim Y before"=w505, "final filter coeff X"=w503, "final filter coeff Y"=w501, "final filter coeff Z"=w499, "final filter coeff X before"=w497, "final filter coeff Y before"=w495, "final filter coeff Z before"=w493, "activate COMx"=w491, "activate COMy"=w490, "activate COMz"=w489, "frequency (periods/tick)"=w485, "duty cycle (periods)"=w488, "amplitude"=w483, "offset"=w484, "pz?"=w482, "eom sine frequency (periods/tick)"=w475, "Amplitude_sine_EOM"=w476, "Big Number"="Big Number", "No_integral_gain"=w469, "Y_emergency_threshould"=w471, "X_emergency_threshould"=w470, "Reset z accum"=w468, "Reset y accum"=w467, "Reset x accum"=w466, "Notch coeff x"=w465, "Notch coeff y 1"=w430, "Notch coeff y 2"=w431, "phase offset AO4"=w421, "frequency AO4"=w428, "reset AO4"=w424, "phase offset AO5"=w415, "frequency AO5"=w412, "reset AO5"=w409, "phase offset AO6"=w420, "frequency AO6"=w427, "reset AO6"=w423, "phase offset AO7"=w414, "frequency AO7"=w411, "reset AO7"=w408, "Amplitude AO4"=w418, "Amplitude AO5"=w406, "Amplitude AO6"=w417, "Amplitude AO7"=w405) -> ("FPGA VI Reference Out"=w613:refnum<k20>, "error out"=w614:errorcluster)  [unwired: 2 in, 2 out]
      }
    }
    n156 = feedback-in #1(w79) -> ()
    n157 = feedback-in #2(w74) -> ()
    n158 = xnode "Read/Write Control"("FPGA VI Reference In"=w128, "error in"=w129) -> ("FPGA VI Reference Out"=w127:refnum<k20>, "error out"=w126:errorcluster, "EOM_amplitude"=w125:i16)
    n159 = case shown="False" "Write data to buffers" {
      tunnel: "Buffer file path" -> [_ w333]
      tunnel: w127 -> [w322 w332]
      tunnel: w126 -> [w321 w331]
      tunnel: [w322 w324] -> w193
      tunnel: [w321 w323] -> w192
      frame False {
      }
      frame True {
        n160 = flat-sequence {
          tunnel: w333 -> [w352]
          tunnel: w332 -> [w350]
          tunnel: w331 -> [w349]
          tunnel: [w344] -> w330
          tunnel: [w343] -> w329
          tunnel: [w337] -> w328
          tunnel: [w342] -> w327
          tunnel: w330 -> [w358]
          tunnel: w329 -> [w357]
          tunnel: w328 -> [w356]
          tunnel: w327 -> [w355]
          tunnel: [w354] -> w326
          tunnel: [w353] -> w325
          tunnel: w326 -> [w400]
          tunnel: w325 -> [w399]
          tunnel: [w398] -> w324
          tunnel: [w397] -> w323
          frame #0 {
            w342 = 0
            n161 = call-poly <vilib>:"Read From Spreadsheet File.vi"("delimiter (\\t)"="," ("delimiter (\\t)"), "format (%d)"="%d", "file path (dialog if empty)"=w352) -> ("all rows"=w337:i64[][])  [unwired: 4 in, 4 out]
            n162 = Index Array(array=w337, index (row)=0, index (col)=0 ("disabled index (col)")) -> (element=w341:i64)
            n163 = Index Array(array=w337, index (row)=0, index (col)=1 ("disabled index (col)")) -> (element=w340:i64)
            n164 = Index Array(array=w337, index (row)=0, index (col)=2 ("disabled index (col)")) -> (element=w334:i64)
            n165 = xnode "Read/Write Control"("FPGA VI Reference In"=w350, "error in"=w349, "data_buffer_1"=w341, "data_buffer2"=w340, "write_address"=w342, "data_buffer3"=w334, "ready_to_write"=TRUE) -> ("FPGA VI Reference Out"=w343:refnum<k20>, "error out"=w344:errorcluster)
          }
          frame #1 {
            n166 = while {
              shift-right: [w359] -> _
              shift-left: w355 -> [w367]
              tunnel: w357 -> [w371]
              tunnel: w358 -> [w370]
              tunnel: w356 -> [w366]
              tunnel: [w361] -> w354
              tunnel: [w360] -> w353
              stop <- w362 stop-if-true
              n167 = xnode "Read/Write Control"("FPGA VI Reference In"=w371, "error in"=w370) -> ("FPGA VI Reference Out"=w365:refnum<k20>, "error out"=w364:errorcluster, "written_address"=w369:u32)
              n168 = Equal?(x=w367, y=w369) -> (x = y?=w368:bool)
              n169 = case shown="True" w368 {
                tunnel: w367 -> [w374 w381]
                tunnel: w366 -> [_ w380]
                tunnel: w365 -> [w373 w379]
                tunnel: w364 -> [w372 w378]
                tunnel: [w374 w377] -> w359
                tunnel: [w373 w376] -> w361
                tunnel: [w372 w375] -> w360
                frame False {
                }
                frame True {
                  n170 = flat-sequence {
                    tunnel: w381 -> [w394]
                    tunnel: w380 -> [w384]
                    tunnel: w379 -> [w391]
                    tunnel: w378 -> [w390]
                    tunnel: [w383] -> w377
                    tunnel: [w388] -> w376
                    tunnel: [w387] -> w375
                    frame #0 {
                      n171 = Add(x=w394, y=1) -> (x+y=w383:i32)
                      n172 = Index Array(array=w384, index (row)=w383, index (col)=0 ("disabled index (col)")) -> (element=w386:i64)
                      n173 = Index Array(array=w384, index (row)=w383, index (col)=1 ("disabled index (col)")) -> (element=w389:i64)
                      n174 = Index Array(array=w384, index (row)=w383, index (col)=2) -> (element=w382:i64)
                      n175 = xnode "Read/Write Control"("FPGA VI Reference In"=w391, "error in"=w390, "data_buffer_1"=w386, "data_buffer2"=w389, "write_address"=w383, "data_buffer3"=w382) -> ("FPGA VI Reference Out"=w388:refnum<k20>, "error out"=w387:errorcluster)
                    }
                  }
                }
              }
              n176 = Equal?(x=w359, y=u16 16384) -> (x = y?=w362:bool)
            }
          }
          frame #2 {
            n177 = xnode "Read/Write Control"("FPGA VI Reference In"=w400, "error in"=w399, "ready_to_write"=FALSE) -> ("FPGA VI Reference Out"=w398:refnum<k20>, "error out"=w397:errorcluster)
          }
        }
      }
    }
    n178 = Divide(x=w125, y=i16 3277) -> (x/y=→"EOM_amplitude_out":dbl)
    n179 = xnode "Read/Write Control"("FPGA VI Reference In"=w193, "error in"=w192) -> ("FPGA VI Reference Out"=w88:refnum<k20>, "error out"=w89:errorcluster, "AI X plot"=w92:i16, "fb X plot"=w172:i16, "tot_fb X plot"=→"Tot feedback + DC, X":i16, "AI Y plot"=w91:i16, "fb Y plot"=w168:i16, "tot_fb Y plot"=→"Tot feedback + DC, Y":i16, "AI Z plot"=w106:i16, "fb Z plot"=w105:i16, "tot_fb Z plot"=→"Tot feedback + DC, Z":i16, "AI X before chamber plot"=w103:i16, "AI Y before chamber plot"=w102:i16, "AI Z before chamber plot"=w101:i16, "fb X before chamber plot"=w100:i16, "fb Y before chamber plot"=w99:i16, "fb Z before chamber plot"=w98:i16, "accum out z1"=→"accum out z1":fxp<+/-,37,37>, "accum out z2"=→"accum out z2":fxp<+/-,37,37>)  [unwired: 1 out]
    n180 = case shown="2" "?" {
      tunnel: w92 -> [w275 w276 _]
      tunnel: [w274 w277 w279] -> w176
      tunnel: w103 -> [w273 _ w278]
      frame 0, Default {
        n181 = Bundle("AI X plot"=w275, "AI X before chamber plot"=w273) -> (w274:T3)  [unwired: 1 in]
      }
      frame 2 {
        n182 = Bundle("AI X plot"=w276, "AI X plot"=w276) -> (w277:cluster{"AI X plot":i16, "AI X plot":i16})  [unwired: 1 in]
      }
      frame 1 {
        n183 = Bundle("AI X before chamber plot"=w278, "AI X before chamber plot"=w278) -> (w279:T4)  [unwired: 1 in]
      }
    }
    "AI0" <- w176
    n184 = case shown="2" "?" {
      tunnel: w172 -> [w268 w269 _]
      tunnel: [w267 w270 w272] -> w174
      tunnel: w100 -> [w266 _ w271]
      frame 0, Default {
        n185 = Bundle("fb X plot"=w268, "fb X before chamber plot"=w266) -> (w267:T5)  [unwired: 1 in]
      }
      frame 2 {
        n186 = Bundle("fb X plot"=w269, "fb X plot"=w269) -> (w270:cluster{"fb X plot":i16, "fb X plot":i16})  [unwired: 1 in]
      }
      frame 1 {
        n187 = Bundle("fb X before chamber plot"=w271, "fb X before chamber plot"=w271) -> (w272:T6)  [unwired: 1 in]
      }
    }
    "Individual feedback, X" <- w174
    n188 = case shown="2" "?" {
      tunnel: w91 -> [w260 w262 _]
      tunnel: [w261 w263 w265] -> w165
      tunnel: w102 -> [w259 _ w264]
      frame 0, Default {
        n189 = Bundle("AI Y plot"=w260, "AI Y before chamber plot"=w259) -> (w261:T7)  [unwired: 1 in]
      }
      frame 2 {
        n190 = Bundle("AI Y plot"=w262, "AI Y plot"=w262) -> (w263:cluster{"AI Y plot":i16, "AI Y plot":i16})  [unwired: 1 in]
      }
      frame 1 {
        n191 = Bundle("AI Y before chamber plot"=w264, "AI Y before chamber plot"=w264) -> (w265:T8)  [unwired: 1 in]
      }
    }
    "AI1" <- w165
    n192 = case shown="2" "?" {
      tunnel: w168 -> [w253 w255 _]
      tunnel: [w254 w256 w258] -> w167
      tunnel: w99 -> [w252 _ w257]
      frame 0, Default {
        n193 = Bundle("fb Y plot"=w253, "fb Y before chamber plot"=w252) -> (w254:T9)  [unwired: 1 in]
      }
      frame 2 {
        n194 = Bundle("fb Y plot"=w255, "fb Y plot"=w255) -> (w256:cluster{"fb Y plot":i16, "fb Y plot":i16})  [unwired: 1 in]
      }
      frame 1 {
        n195 = Bundle("fb Y before chamber plot"=w257, "fb Y before chamber plot"=w257) -> (w258:T10)  [unwired: 1 in]
      }
    }
    "Individual feedback, Y" <- w167
    n196 = case shown="2" "?" {
      tunnel: w106 -> [w228 w230 _]
      tunnel: [w229 w231 w233] -> w107
      tunnel: w101 -> [w227 _ w232]
      frame 0, Default {
        n197 = Bundle("AI Z plot"=w228, "AI Z before chamber plot"=w227) -> (w229:T11)  [unwired: 1 in]
      }
      frame 2 {
        n198 = Bundle("AI Z plot"=w230, "AI Z plot"=w230) -> (w231:cluster{"AI Z plot":i16, "AI Z plot":i16})  [unwired: 1 in]
      }
      frame 1 {
        n199 = Bundle("AI Z before chamber plot"=w232, "AI Z before chamber plot"=w232) -> (w233:T12)  [unwired: 1 in]
      }
    }
    "AI 2" <- w107
    n200 = case shown="2" "?" {
      tunnel: w105 -> [w221 w223 _]
      tunnel: [w222 w224 w226] -> w108
      tunnel: w98 -> [w220 _ w225]
      frame 0, Default {
        n201 = Bundle("fb Z plot"=w221, "fb Z before chamber plot"=w220) -> (w222:T13)  [unwired: 1 in]
      }
      frame 2 {
        n202 = Bundle("fb Z plot"=w223, "fb Z plot"=w223) -> (w224:cluster{"fb Z plot":i16, "fb Z plot":i16})  [unwired: 1 in]
      }
      frame 1 {
        n203 = Bundle("fb Z before chamber plot"=w225, "fb Z before chamber plot"=w225) -> (w226:T14)  [unwired: 1 in]
      }
    }
    "Individual feedback, Z" <- w108
  }
  n204 = xnode "Close FPGA VI Reference"("FPGA VI Reference In"=w2, "error in"=w3) -> ("error out"=w8:errorcluster)
  n205 = call <vilib>:"Simple Error Handler.vi"("error in (no error)"=w8) -> ()  [unwired: 4 in, 5 out]
